vi "Path Tuning.vi"(6 "Tune":bool[](array[boolean]), 9 "Measured Position":dbl[](array[numeric]), 10 "Default Y":dbl, 11 "Default X":dbl) -> (3 "Ellipse Length":dbl[](array[numeric]))   [LabVIEW 2021]
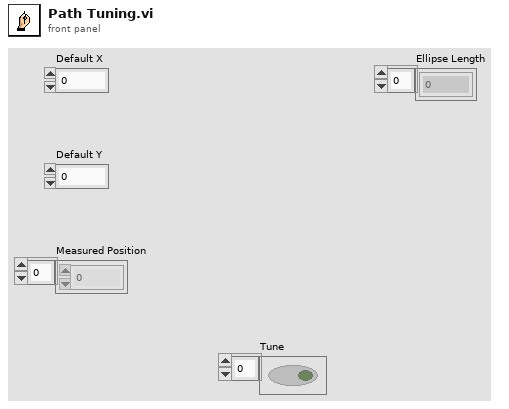
[diagram p1: front panel]
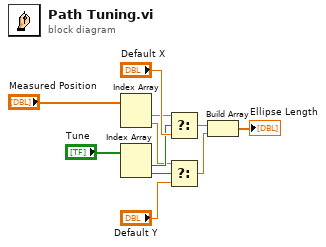
[diagram p0: block diagram]
diagram:
  n1 = Index Array(array="Measured Position") -> (element #1=w2:dbl, element #2=w3:dbl)  [unwired: 2 in]
  n2 = Index Array(array="Tune") -> (element #1=w5:bool, element #2=w6:bool)  [unwired: 2 in]
  n3 = Select(t=w2, s=w5, f="Default X") -> (s? t:f=w9:dbl)
  n4 = Select(t=w3, s=w6, f="Default Y") -> (s? t:f=w10:dbl)
  n5 = Build Array(w9, w10) -> (→"Ellipse Length":dbl[])
